vi "From JSON.vi"(8 "error in (no error)":errorcluster, 10 "JSON In":string, 11 "Boolean in":refnum<class "Abs_Boolean.lvclass">) -> (0 "error out":errorcluster, 3 "Boolean out":refnum<class "Abs_Boolean.lvclass">)   [LabVIEW 2021, in "Abs_Boolean.lvclass"]
uses:
  Abs_Boolean.lvclass
  C:/Program Files (x86)/National Instruments/LabVIEW 2021/vi.lib/TSA/Abstract Data Classes/Abs_Types/Type/Abs_Type.lvclass
  a1a6a1c1-be78-492d-bead-ba3bec5716f1.vi
  <vilib>/JDP Science/JSONtext/Find Item.vi
  <vilib>/JDP Science/JSONtext/Next JSON Value.vi
  <vilib>/JDP Science/JSONtext/String Subset.vi
  <vilib>/JDP Science/JSONtext/Parsing/Advance past next JSON Value (inlined COPY).vi
  <vilib>/JDP Science/JSONtext/Parsing/Advance past whitespace.vi
  <vilib>/JDP Science/JSONtext/Parsing/Advance past String.vi
  <vilib>/JDP Science/JSONtext/Parsing/Advance past Number.vi
  <vilib>/JDP Science/JSONtext/Parsing/Advance past Line Ending.vi
  <vilib>/Utility/LVClass/Get LV Class Name.vi
  <vilib>/JDP Science/JSONtext/Parsing/Parse Full Path or Item Name.vi
  <vilib>/JDP Science/JSONtext/Parsing/Advance past Array.vi
  <vilib>/JDP Science/JSONtext/Parsing/Advance past Object.vi
  <vilib>/JDP Science/JSONtext/support/Error Cluster From Code.vi
  <vilib>/JDP Science/JSONtext/Offset/Find Item Locations by Path.vi
  <vilib>/JDP Science/JSONtext/JSON text to Variant.vi
  <vilib>/JDP Science/JSONtext/LVClass Serializer/JSONtext LVClass Serializer.lvclass
  Value/Abs_Value.lvclass
  Type/Abs_Type.lvclass
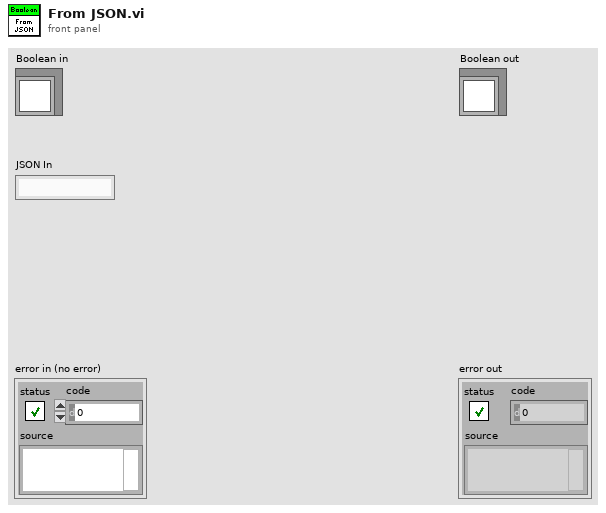
[diagram p1: front panel]
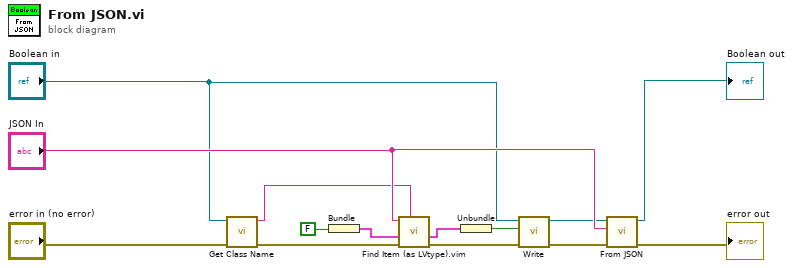
[diagram p0: block diagram]
diagram:
  n1 = call "Get Class Name.vi"("error in (no error)"="error in (no error)", "Abs_Type in"="Boolean in") -> ("error out"=w6:errorcluster, "class name"=w7:string)  [unwired: 8 in]
  n2 = Bundle(FALSE) -> (w8:cluster{bool})  [unwired: 1 in]
  n3 = call "Find Item (as LVtype).vim"("$Path or Item Name"=w7, "error in (no error)"=w6, "Data Type and Default Value"=w8, "JSON"="JSON In") -> ("error out"=w5:errorcluster, "Data"=w9:cluster{bool})  [unwired: 4 in, 2 out]
  n4 = Unbundle(w9) -> (w2:bool)
  n5 = call-dynamic "Write.vi"("error in (no error)"=w5, "Boolean"=w2, "Boolean in"="Boolean in") -> ("error out"=w4:errorcluster, "Boolean out"=w3:refnum<class "Abs_Boolean.lvclass">)  [unwired: 7 in]
  n6 = call-parent "From JSON.vi"("error in (no error)"=w4, "JSON"="JSON In", "Type in"=w3) -> ("error out"=→"error out":errorcluster, "Type out"=→"Boolean out":refnum<class "Abs_Boolean.lvclass">)  [unwired: 7 in]
